vi "main.vi"() -> ()   [LabVIEW 2011]
panel:
  in  "Array":timestamp[](array[timestamp])
  out "Array 2":dbl[](array[numeric])
  in  "Instances":i32
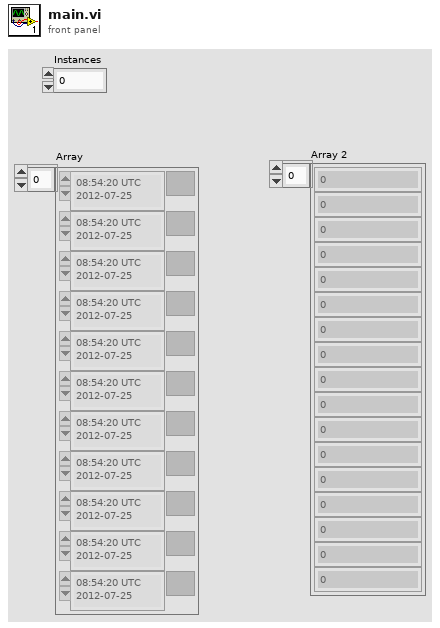
[diagram p1: front panel]
types:
  T1 = typedef "Semaphore RefNum" = refnum<k1>
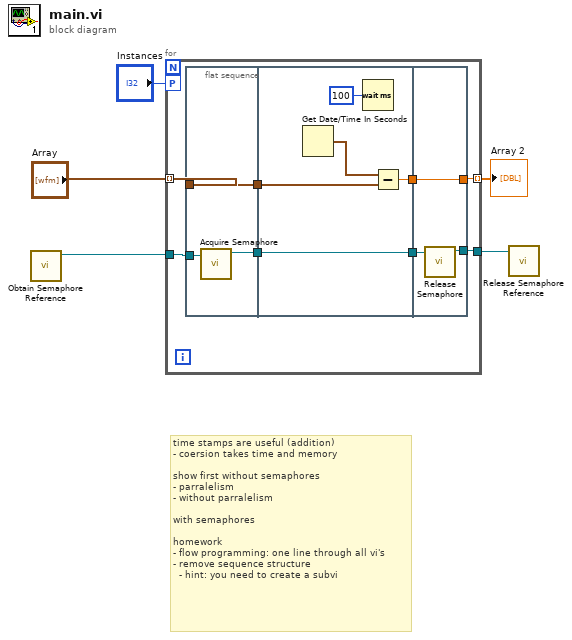
[diagram p0: block diagram]
diagram:
  # "time stamps are useful (addition)\n- coersion takes time and memory\n\nshow first without semaphores\n- parralelism\n- without parralelism\n\nwith semaphores\n\nhomework\n- flow programming: one line through all vi's\n- remove sequence structure\n  - hint: you need to create a subvi"
  n1 = call <vilib>:"Obtain Semaphore Reference.vi"() -> ("semaphore"=w2:T1)  [unwired: 5 in, 2 out]
  n2 = for {
    workers-P: "Instances" -> [_]
    tunnel: "Array" -> [w13] mode=indexing
    tunnel: [w12] -> w4 mode=indexing
    tunnel: w2 -> [w10]
    tunnel: [w6] -> w1
    n3 = flat-sequence {
      tunnel: w13 -> [w16]
      tunnel: [w16] -> w11
      tunnel: w10 -> [w15]
      tunnel: [w14] -> w9
      tunnel: w11 -> [w19]
      tunnel: w9 -> [w17]
      tunnel: [w18] -> w8
      tunnel: [w17] -> w7
      tunnel: [w24] -> w12
      tunnel: w8 -> [w24]
      tunnel: w7 -> [w23]
      tunnel: [w22] -> w6
      frame #0 {
        n4 = call <vilib>:"Acquire Semaphore.vi"("semaphore"=w15) -> ("semaphore out"=w14:T1)  [unwired: 4 in, 2 out]
      }
      frame #1 {
        n5 = Get Date/Time In Seconds() -> (seconds since 1Jan1904=w20:timestamp)
        n6 = Wait (ms)(milliseconds to wait=u32 100) -> ()  [unwired: 1 out]
        n7 = Subtract(x=w20, y=w19) -> (x-y=w18:dbl)
      }
      frame #2 {
        n8 = call <vilib>:"Release Semaphore.vi"("semaphore"=w23) -> ("semaphore out"=w22:T1)  [unwired: 5 in, 1 out]
      }
    }
  }
  "Array 2" <- w4
  n9 = call <vilib>:"Release Semaphore Reference.vi"("semaphore"=w1) -> ()  [unwired: 9 in, 2 out]
